vi "Analyse error.vi"(8 "error in (no error)":errorcluster, 11 "ErrorHandler JSON in":refnum<class "ErrorHandler JSON.lvclass">) -> (0 "error out":errorcluster, 3 "ErrorHandler JSON out":refnum<class "ErrorHandler JSON.lvclass">)   [LabVIEW 2020, in "wamplv.lvlib" / "ErrorHandler JSON.lvclass"]
uses:
  ErrorHandler JSON.lvclass
  ErrorHandler JSON.lvclass/ErrorHandler JSON.ctl
  <vilib>/ErrorRing/Error Ring.xnode
  <vilib>/Utility/error.llb/Error Cluster From Error Code.vi
  wamplv.lvlib
  Utils/Utils.lvclass
  SerialisedMessages/JSONMessage/WampMessage JSON.lvclass
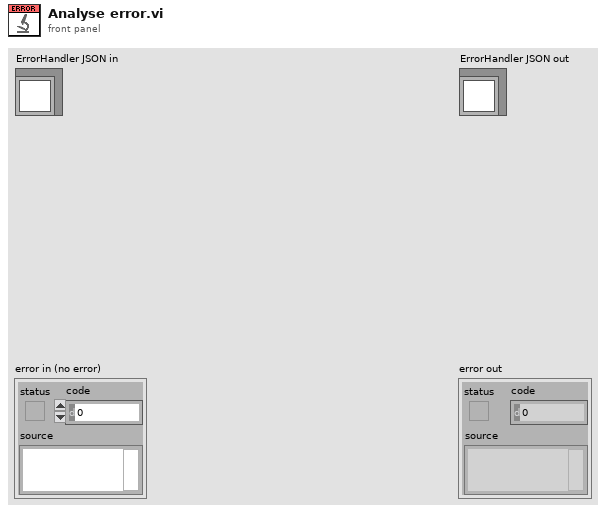
[diagram p1: front panel]
types:
  T1 = typedef "wamplv.lvlib/WAMP Message Codes.ctl" = enum8{"HELLO", "WELCOME", "CHALLENGE", "AUTHENTICATE", "ABORT", "GOODBYE", "ERROR", "PUBLISH", "PUBLISHED", "SUBSCRIBE", "SUBSCRIBED", "UNSUBSCRIBE", "UNSUBSCRIBED", "EVENT", "CALL", "RESULT", "REGISTER", "REGISTERED", "UNREGISTER", "UNREGISTERED", "INVOCATION", "YIELD"}
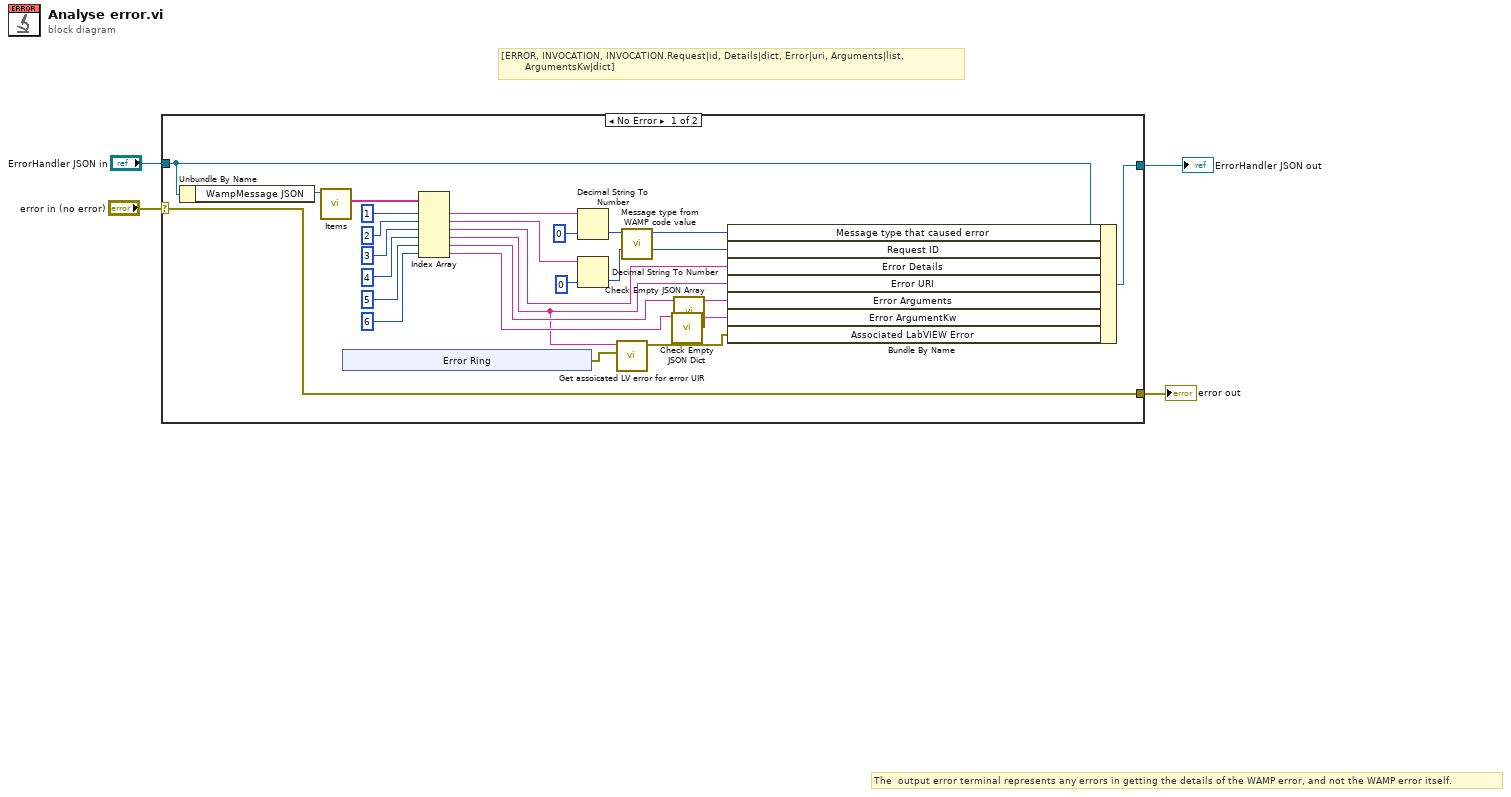
[diagram p0: block diagram]
diagram:
  # "[ERROR, INVOCATION, INVOCATION.Request|id, Details|dict, Error|uri, Arguments|list,\n        ArgumentsKw|dict]"
  # "The  output error terminal represents any errors in getting the details of the WAMP error, and not the WAMP error itself."
  n1 = case shown="No Error" "error in (no error)" {
    selector: "error in (no error)" -> [w5 w36]
    tunnel: "ErrorHandler JSON in" -> [w7 w35]
    tunnel: [w5 w36] -> w2
    tunnel: [w30 w35] -> w1
    frame No Error {
      n2 = Unbundle By Name(w7) -> ("WampMessage JSON"=w6:refnum<class "WampMessage JSON.lvclass">)
      n3 = call-dynamic "Items.vi"("JSONMessage in"=w6) -> ("<JSON>Elements"=w28:string[])  [unwired: 9 in, 1 out]
      n4 = xnode "Error Ring"() -> ("error out"=w8:errorcluster)
      n5 = Index Array(array=w28, index #1=1 ("index"), index #2=2 ("index"), index #3=3 ("index"), index #4=4 ("index"), index #5=5 ("index"), index #6=6 ("index")) -> (element #1=w23:string, element #2=w18:string, element #3=w16:string, element #4=w10:string, element #5=w12:string, element #6=w13:string)
      n6 = Decimal String To Number(string=w23, default (0L)=u8 0 ("WAMP Numeric value")) -> (number=w21:u8)  [unwired: 1 in, 1 out]
      n7 = Decimal String To Number(string=w18, default (0L)=u64 0 ("Error data (JSON).Request ID")) -> (number=w17:u64)  [unwired: 1 in, 1 out]
      n8 = call "Get assoicated LV error for error UIR.vi"("Default error"=w8, "URI"=w10) -> ("Associated error"=w9:errorcluster)  [unwired: 9 in]
      n9 = call "Message type from WAMP code value.vi"("WAMP Numeric value"=w21) -> ("Message Type"=w20:T1)  [unwired: 7 in, 1 out]
      n10 = call "Check Empty JSON Dict.vi"("JSON in"=w13) -> ("JSON out"=w14:string)  [unwired: 10 in]
      n11 = call "Check Empty JSON Array.vi"("JSON in"=w12) -> ("JSON out"=w11:string)  [unwired: 10 in]
      n12 = Bundle By Name(cluster=w7, "Message type that caused error"=w20, "Request ID"=w17, "Error Details"=w16, "Error URI"=w10, "Error Arguments"=w11, "Error ArgumentKw"=w14, "Associated LabVIEW Error"=w9) -> (w30:refnum<class "ErrorHandler JSON.lvclass">)
    }
    frame Error {
    }
  }
  "error out" <- w2
  "ErrorHandler JSON out" <- w1
